vi "comm get handles.vi"(8 "error in (no error)":errorcluster) -> (0 "error out":errorcluster, 3 "handles":u64[](array[numeric]))   [LabVIEW 2009, in "lvserial.lvlib"]
doc: "This function returns the handles of all actually opened serial ports."
uses:
  lvserial.lvlib
  x64/Release/lvserial.dll
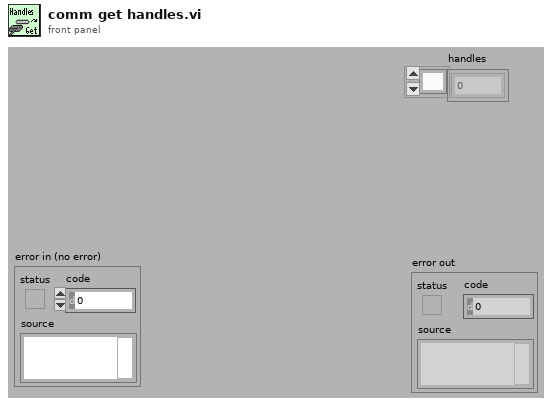
[diagram p1: front panel]
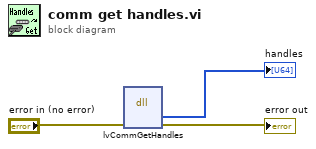
[diagram p0: block diagram]
diagram:
  n1 = dll-call lib="C:/Users/Admin/Desktop/lvserial_source_1-2-13/x64/Release/lvserial.dll" fn="lvCommGetHandles"("pError"="error in (no error)") -> ("phaulHandles"=→"handles":u64[], "pError"=→"error out":errorcluster)  [unwired: 3 in, 4 out]
